vi "Temp.vi"() -> ()   [LabVIEW 2024, in "Flexi-Flow Modbus TCP API.lvlib"]
uses:
  Flexi-Flow Modbus TCP API.lvlib
  <vilib>/Plasmionique/MB Master/MB_Master_TCP/MB_Master_TCP.lvclass
  <vilib>/Plasmionique/MB Master/MB Master.lvlib
panel:
  in  "IP Address":string="192.168.100.10"
  in  "value":u16
  in  "address":u16
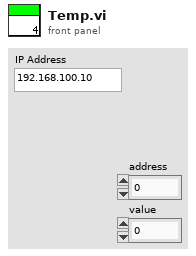
[diagram p1: front panel]
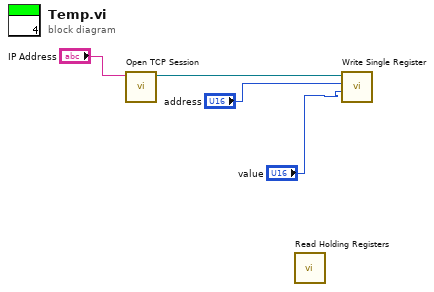
[diagram p0: block diagram]
diagram:
  n1 = call <vilib>:"Open TCP Session.vi"("IP Address"="IP Address") -> ("MB_TCP session"=w3:refnum<class "MB_Master_TCP.lvclass">)  [unwired: 9 in, 1 out]
  n2 = call <vilib>:"Read Holding Registers.vi"() -> ()  [unwired: 9 in, 3 out]
  n3 = call <vilib>:"Write Single Register.vi"("value"="value", "address"="address", "MB session in"=w3) -> ()  [unwired: 7 in, 2 out]
